vi "TestMain.vi"   [LabVIEW 2017]
uses:
  Login-UI.lvlib
types:
  T1 = cluster{"HideMain(T)":bool, "RetryAllowed(T)":bool}
  T2 = typedef "Login-UI.lvlib/User-Info.ctl" = cluster{"UserName":string, "Password":string, "Role":T3}
  T3 = typedef "Login-UI.lvlib/User-Role.ctl" = enum16{"INVALID", "Operator", "Engineer", "Admin"}
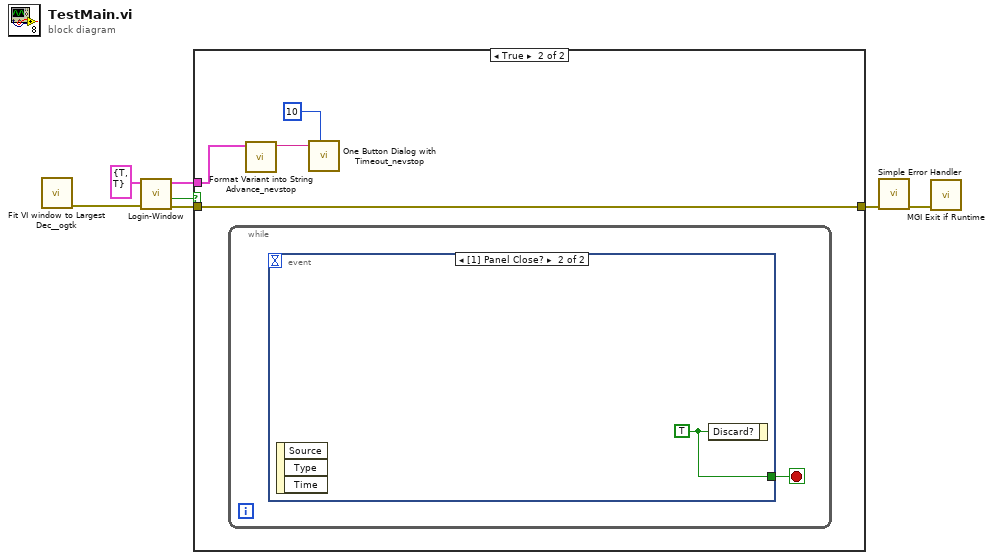
[diagram p0: block diagram]
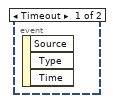
[diagram p3: hidden frame]
diagram:
  n1 = call <userlib>:"Fit VI window to Largest Dec__ogtk.vi"() -> ("error out"=w2:errorcluster)  [unwired: 6 in, 1 out]
  n2 = call "Login-Window.vi"("Error in"=w2, "Options"=T1 {"HideMain(T)"=TRUE, "RetryAllowed(T)"=TRUE}) -> ("Error out"=w4:errorcluster, "Valid User"=w6:bool, "User Info"=w5:T2)  [unwired: 7 in]
  n3 = case shown="True" w6 {
    tunnel: w5 -> [_ w12]
    tunnel: w4 -> [w8 w9]
    tunnel: [w8 w9] -> w3
    frame False {
    }
    frame True {
      n4 = while {
        stop <- w13 stop-if-true
        n5 = event shown="[1] Panel Close?" {
          selector: _ -> [_ _]
          dyn-events: _ -> [_ _]
          timeout: _ -> [_ _]
          tunnel: [_ w14] -> w13
          event Timeout {
            n6 = event-data() -> ()  [unwired: 1 in, 3 out]
          }
          event Panel Close? {
            w14 = TRUE ("Discard?")
            n7 = event-data() -> ()  [unwired: 1 in, 3 out]
            n8 = event-data("Discard?"=w14) -> ()  [unwired: 1 in, 1 out]
          }
        }
      }
      n9 = call <userlib>:"Format Variant into String Advance_nevstop.vi"("Variant"=w12) -> ("Data"=w11:string)  [unwired: 8 in, 2 out]
      n10 = call <userlib>:"One Button Dialog with Timeout_nevstop.vi"("message"=w11, "Btn Timeout(-1 s)"=10) -> ()  [unwired: 7 in, 1 out]
    }
  }
  n11 = call <vilib>:"Simple Error Handler.vi"("error in (no error)"=w3) -> ("error out"=w7:errorcluster)  [unwired: 4 in, 4 out]
  n12 = call <userlib>:"MGI Exit if Runtime.vi"("Error In (Dependency Only)"=w7) -> ()  [unwired: 11 in]
